vi "Cleanup.vi"(8 "error in (no error)":errorcluster, 11 "User Provider in":refnum<class "User Provider.lvclass">) -> (0 "error out":errorcluster)   [LabVIEW 2020, in "HTTP Server.lvlib" / "User Provider.lvclass"]
uses:
  User Provider.lvclass
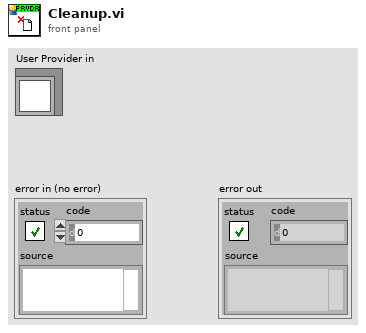
[diagram p1: front panel]
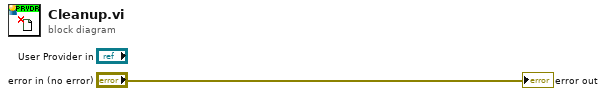
[diagram p0: block diagram]
diagram:
  "error out" <- "error in (no error)"
